vi "StoreFrontPanelSettings.vi"(8 "error in (no error)":errorcluster, 11 "AutoModeData in":T1) -> (0 "error out":errorcluster, 3 "AutoModeData out":T1)   [LabVIEW 2019, in "AutoMode.lvlib"]
uses:
  AutoMode.lvlib
  Cluster - AutoModeData.ctl
  MainController/Cluster - TestSettings.ctl
  MainController/Cluster - HardwareConfiguration.ctl
  MainController/Cluster - TestResults.ctl
  Cluster - AutoModeMessage.ctl
  Enum - AutoModeState.ctl
  MainController/Cluster - MainControllerMessage.ctl
  MainController/Enum - MainState.ctl
  <vilib>/Utility/config.llb/Write Key (I32).vi
  <vilib>/Utility/config.llb/Write Key (U32).vi
  <vilib>/Utility/config.llb/Write Key (String).vi
  <vilib>/Utility/config.llb/Write Key (Path).vi
  <vilib>/Utility/config.llb/Write Key (Double).vi
  <vilib>/Utility/config.llb/Write Key (Boolean).vi
  <vilib>/Utility/config.llb/NI_LVConfig.lvlib
  <vilib>/Utility/Data Type/NI_Data Type.lvlib
  MainController/MainController.lvlib
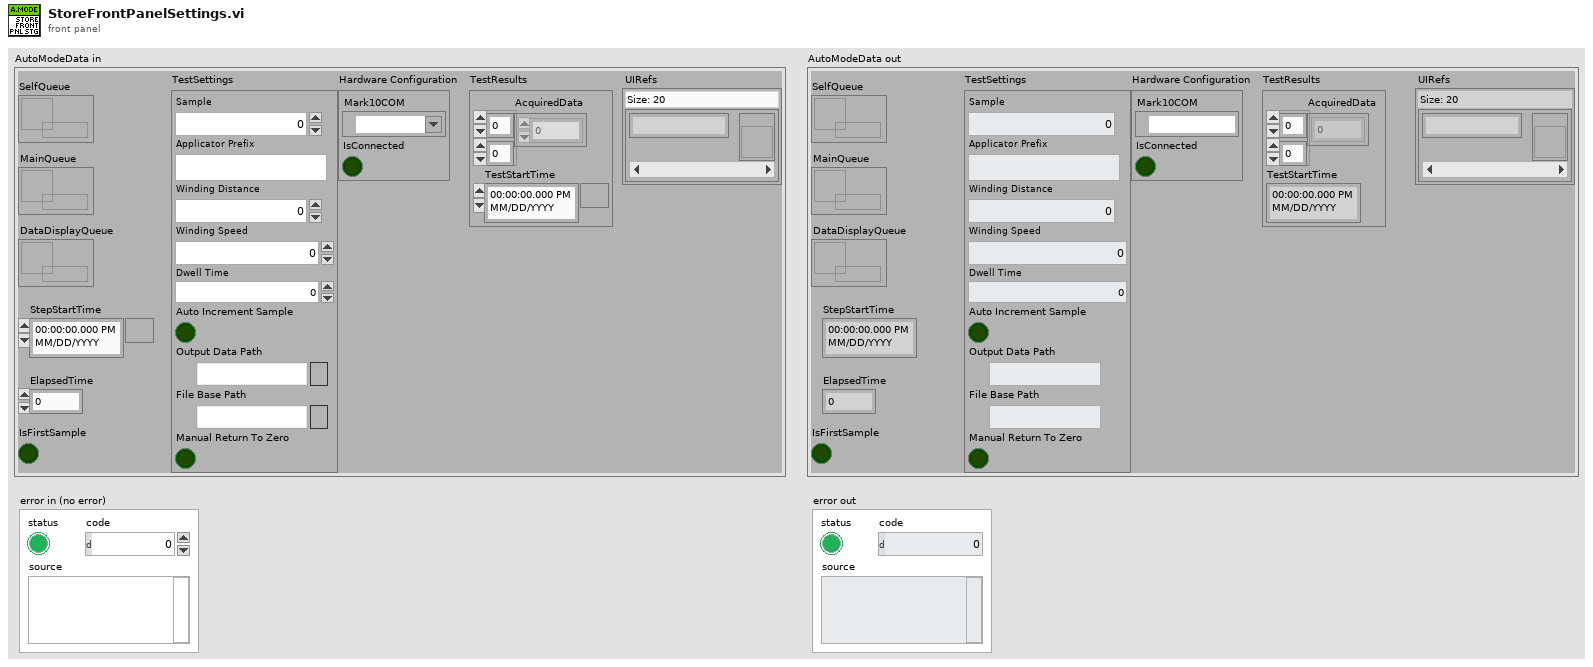
[diagram p1: front panel]
types:
  T1 = typedef "AutoMode.lvlib/Cluster - AutoModeData.ctl" = cluster{"DataDisplayQueue":refnum<queue>, "StepStartTime":timestamp, "TestSettings":T2, "Hardware Configuration":T3, "TestResults":T4, "ElapsedTime":dbl, "IsFirstSample":bool, "SelfQueue":refnum<queue>, "MainQueue":refnum<queue>, "UIRefs":map{string, refnum<vi>}}
  T2 = typedef "MainController.lvlib/Cluster - TestSettings.ctl" = cluster{"Sample":u32, "Applicator Prefix":string, "Winding Distance":dbl, "Winding Speed":dbl, "Dwell Time":dbl, "Auto Increment Sample":bool, "Output Data Path":path, "File Base Path":path, "Manual Return To Zero":bool}
  T3 = typedef "MainController.lvlib/Cluster - HardwareConfiguration.ctl" = cluster{"Mark10COM":refnum<visa-resource-name>, "IsConnected":bool}
  T4 = typedef "MainController.lvlib/Cluster - TestResults.ctl" = cluster{"AcquiredData":dbl[][], "TestStartTime":timestamp}
  T5 = typedef "NI_LVConfig.lvlib/Config Data RefNum.ctl" = refnum<k1>
  T6 = typedef "NI_Data Type.lvlib/Data Type.ctl" = enum8{"Invalid Type", "Void", "I8", "I16", "I32", "I64", "U8", "U16", "U32", "U64", "Single Float", "Double Float", "Extended Float", "Single Complex", "Double Complex", "Extended Complex", "Enum U8", "Enum U16", "Enum U32", "Enum U64", "Single Float With Unit", "Double Float With Unit", "Extended Float With Unit", "Single Complex with Unit", "Double Complex with Unit", "Extended Complex with Unit", "Boolean", "String", "Path", "Picture", "Tag", "Array", "Cluster", "Variant", "LV Variant", "Waveform", "Timestamp", "Digital Waveform", "Digital Data", "ExpressData", "Refnum", "External Data", "VI", "Poly VI", "LabVIEW Class Instance", "Fixed Point", "Set Collection", "Map Collection"}
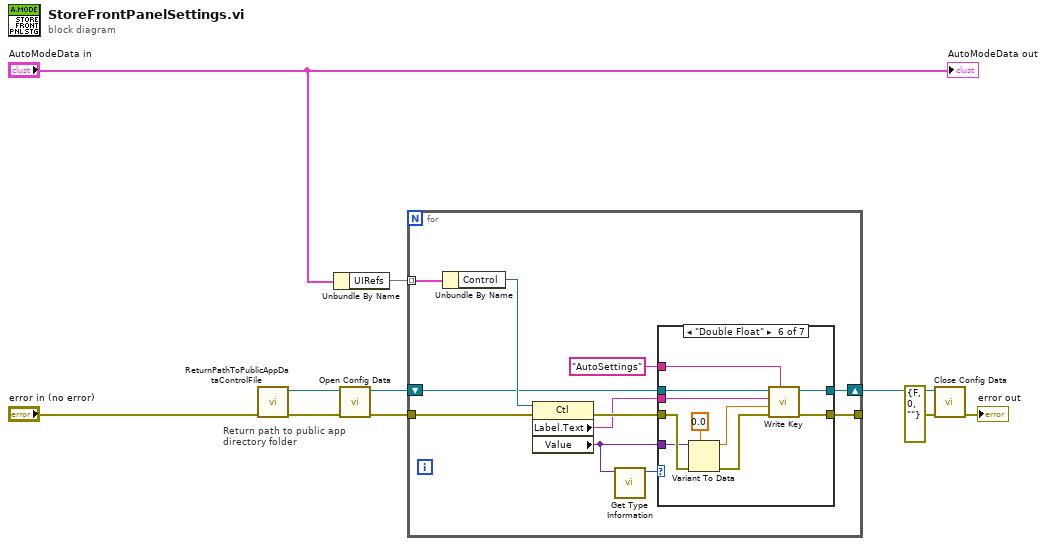
[diagram p0: block diagram]
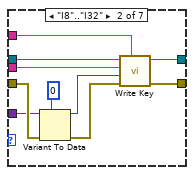
[diagram p3: hidden frame]
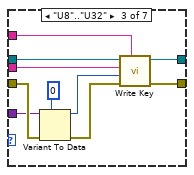
[diagram p4: hidden frame]
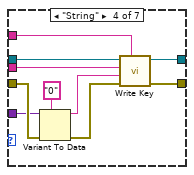
[diagram p5: hidden frame]
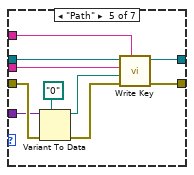
[diagram p6: hidden frame]
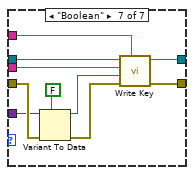
[diagram p7: hidden frame]
diagram:
  # "Return path to public app directory folder"
  n1 = call "ReturnPathToPublicAppDataControlFile.vi"("error in (no error)"="error in (no error)") -> ("error out"=w8:errorcluster, "UIControlsFilePath"=w6:path)  [unwired: 9 in]
  n2 = Unbundle By Name("AutoModeData in") -> ("UIRefs"=w9:map{string, refnum<vi>})
  n3 = call <vilib>:"Open Config Data.vi"("error in (no error)"=w8, "configuration file path"=w6) -> ("error out"=w3:errorcluster, "refnum"=w4:T5)  [unwired: 7 in, 1 out]
  n4 = for {
    tunnel: w9 -> [w21] mode=indexing
    shift-right: [w11] -> w2
    shift-left: w4 -> [w14]
    tunnel: w3 -> [w19]
    tunnel: [w16] -> _
    n5 = Unbundle By Name(w21) -> ("Control"=w20:refnum<vi>)
    n6 = property class="Ctl"(reference=w20, error in=w19) -> (error out=w15:errorcluster, "Label.Text"=w13:string, "Value"=w17:variant)  [unwired: 1 out]
    n7 = call <vilib>:"Get Type Information.vi"("variant"=w17) -> ("type"=w18:T6)  [unwired: 6 in, 4 out]
    n8 = case shown="\"Double Float\"" w18 {
      tunnel: w17 -> [_ w31 w41 w51 w61 w71 w81]
      tunnel: [w23 w29 w39 w49 w59 w69 w79] -> w16
      tunnel: w15 -> [w23 w33 w43 w53 w63 w73 w83]
      tunnel: w14 -> [w22 w28 w38 w48 w58 w68 w78]
      tunnel: w13 -> [_ w27 w37 w47 w57 w67 w77]
      tunnel: "AutoSettings" ("section") -> [_ w26 w36 w46 w56 w66 w76]
      tunnel: [w22 w24 w34 w44 w54 w64 w74] -> w11
      frame Default {
      }
      frame "I8".."I32" {
        n9 = Variant To Data(error in=w33, type=0, Variant=w31) -> (data=w25:i32, error out=w32:errorcluster)
        n10 = call-poly <vilib>:"Write Key.vi"("section"=w26, "error in (no error)"=w32, "value"=w25, "key"=w27, "refnum"=w28) -> ("error out"=w29:errorcluster, "refnum out"=w24:T5)  [unwired: 4 in, 1 out]
      }
      frame "U8".."U32" {
        n11 = Variant To Data(error in=w43, type=u32 0, Variant=w41) -> (data=w35:u32, error out=w42:errorcluster)
        n12 = call-poly <vilib>:"Write Key.vi"("section"=w36, "error in (no error)"=w42, "value"=w35, "key"=w37, "refnum"=w38) -> ("error out"=w39:errorcluster, "refnum out"=w34:T5)  [unwired: 4 in, 1 out]
      }
      frame "String" {
        n13 = Variant To Data(error in=w53, type="0", Variant=w51) -> (data=w45:string, error out=w52:errorcluster)
        n14 = call-poly <vilib>:"Write Key.vi"("section"=w46, "error in (no error)"=w52, "value"=w45, "key"=w47, "refnum"=w48) -> ("error out"=w49:errorcluster, "refnum out"=w44:T5)  [unwired: 4 in, 1 out]
      }
      frame "Path" {
        n15 = Variant To Data(error in=w63, type=path "0", Variant=w61) -> (data=w55:path, error out=w62:errorcluster)
        n16 = call-poly <vilib>:"Write Key.vi"("section"=w56, "error in (no error)"=w62, "value"=w55, "key"=w57, "refnum"=w58) -> ("error out"=w59:errorcluster, "refnum out"=w54:T5)  [unwired: 4 in, 1 out]
      }
      frame "Double Float" {
        n17 = Variant To Data(error in=w73, type=0.0, Variant=w71) -> (data=w65:dbl, error out=w72:errorcluster)
        n18 = call-poly <vilib>:"Write Key.vi"("section"=w66, "error in (no error)"=w72, "value"=w65, "key"=w67, "refnum"=w68) -> ("error out"=w69:errorcluster, "refnum out"=w64:T5)  [unwired: 4 in, 1 out]
      }
      frame "Boolean" {
        n19 = Variant To Data(error in=w83, type=FALSE, Variant=w81) -> (data=w75:bool, error out=w82:errorcluster)
        n20 = call-poly <vilib>:"Write Key.vi"("section"=w76, "error in (no error)"=w82, "value"=w75, "key"=w77, "refnum"=w78) -> ("error out"=w79:errorcluster, "refnum out"=w74:T5)  [unwired: 4 in, 1 out]
      }
    }
  }
  n21 = call <vilib>:"Close Config Data.vi"("error in (no error)"=errorcluster {"status"=FALSE, "code"=0, "source"=""}, "refnum"=w2) -> ("error out"=→"error out":errorcluster)  [unwired: 8 in, 1 out]
  "AutoModeData out" <- "AutoModeData in"
